vi "startReadUntilIntensity.vi"(8 "error in (no error)":errorcluster, 9 "ElectrometerController in":refnum<class "ElectrometerController.lvclass">, 10 "Intensity":dbl format="%#_13g", 11 "ReadyState in":refnum<class "ReadyState.lvclass">) -> (0 "error out":errorcluster, 1 "ElectrometerController out":refnum<class "ElectrometerController.lvclass">, 3 "ReadyState out":refnum<class "ReadyState.lvclass">)   [LabVIEW 2016, in "ReadyState.lvclass"]
uses:
  ReadyState.lvclass
  ElectrometerController/ElectrometerController.lvclass
  internalState.ctl
  ElectrometerState.lvclass
  Electrometer.lvclass
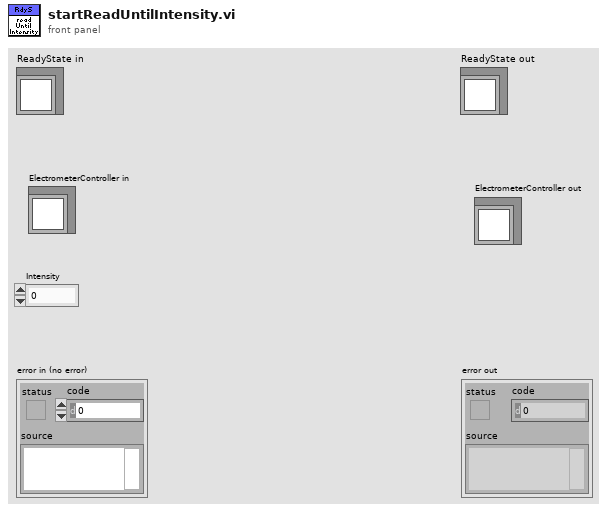
[diagram p1: front panel]
types:
  T1 = typedef "Electrometer.lvclass/internalState.ctl" = enum16{"Ready", "Configuring", "ManualReading", "UntilIntensityReading", "SetDurationReading"}
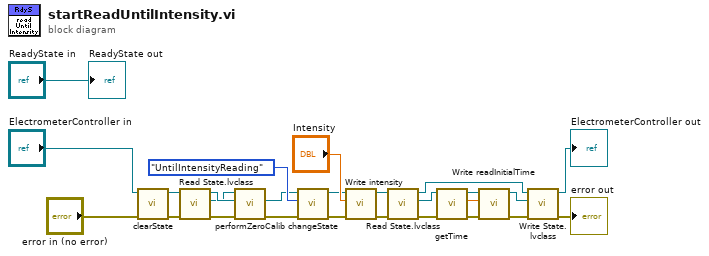
[diagram p0: block diagram]
diagram:
  n1 = call "clearState.vi"("error in (no error)"="error in (no error)", "ElectrometerController in"="ElectrometerController in") -> ("error out"=w1:errorcluster, "ElectrometerController out"=w2:refnum<class "ElectrometerController.lvclass">)  [unwired: 8 in]
  n2 = call-dynamic "Read State.lvclass.vi"("error in (no error)"=w1, "ElectrometerController in"=w2) -> ("error out"=w20:errorcluster, "ElectrometerState"=w18:refnum<class "ElectrometerState.lvclass">, "ElectrometerController out"=w19:refnum<class "ElectrometerController.lvclass">)  [unwired: 7 in]
  n3 = call-dynamic "performZeroCalib.vi"("error in (no error)"=w20, "ElectrometerController in"=w19, "State in"=w18) -> ("error out"=w14:errorcluster, "ElectrometerController out"=w15:refnum<class "ElectrometerController.lvclass">)  [unwired: 5 in, 2 out]
  n4 = call "changeState.vi"("error in (no error)"=w14, "State"=internalState."UntilIntensityReading", "ElectrometerController in"=w15) -> ("error out"=w12:errorcluster, "ElectrometerController out"=w13:refnum<class "ElectrometerController.lvclass">)  [unwired: 7 in]
  n5 = call-dynamic "Write intensity.vi"("error in (no error)"=w12, "intensity"="Intensity", "ElectrometerController in"=w13) -> ("error out"=w11:errorcluster, "ElectrometerController out"=w10:refnum<class "ElectrometerController.lvclass">)  [unwired: 7 in]
  n6 = call-dynamic "Read State.lvclass.vi"("error in (no error)"=w11, "ElectrometerController in"=w10) -> ("error out"=w9:errorcluster, "ElectrometerState"=w8:refnum<class "ElectrometerState.lvclass">, "ElectrometerController out"=w7:refnum<class "ElectrometerController.lvclass">)  [unwired: 7 in]
  n7 = call-dynamic "getTime.vi"("error in (no error)"=w9, "State in"=w8) -> ("error out"=w22:errorcluster, "relative seconds"=w23:dbl, "State out"=w21:refnum<class "ElectrometerState.lvclass">)  [unwired: 7 in]
  n8 = call-dynamic "Write readInitialTime.vi"("error in (no error)"=w22, "readInitialTime"=w23, "State in"=w21) -> ("error out"=w24:errorcluster, "State out"=w25:refnum<class "ElectrometerState.lvclass">)  [unwired: 7 in]
  n9 = call-dynamic "Write State.lvclass.vi"("error in (no error)"=w24, "ElectrometerState"=w25, "ElectrometerController in"=w7) -> ("error out"=→"error out":errorcluster, "ElectrometerController out"=→"ElectrometerController out":refnum<class "ElectrometerController.lvclass">)  [unwired: 7 in]
  "ReadyState out" <- "ReadyState in"
